vi "SysDef.SimpleSave.vi"(8 "error in (no error)":errorcluster, 11 "ID":u64) -> (0 "error out":errorcluster, 3 "ID out":u64)   [LabVIEW 2015, in "System Definition Utilities.lvlib"]
uses:
  System Definition Utilities.lvlib
  _Types/File.DataType.ctl
  _SubVIs/SysDef.Globals.vi
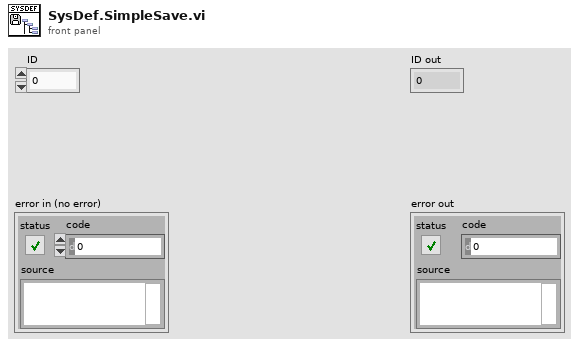
[diagram p1: front panel]
types:
  T1 = typedef "System Definition Utilities.lvlib/SysDef.Export.ctl" = cluster{"Version":string, "Tree":T2[]}
  T2 = typedef "System Definition Utilities.lvlib/TreeItem.ctl" = cluster{"Item Info":T3, "Parent Path":string[], "Properties":T8[]}
  T3 = typedef "System Definition Utilities.lvlib/TreeItem.Info.ctl" = cluster{"Name":string, "Description":string, "GUID":string, "Is Channel":bool, "Channel":T4, "Is Waveform":bool, "Waveform":T6}
  T4 = typedef "Custom Device API.lvlib/Custom Device Channel.ctl" = cluster{"Type":T5, "Units":string, "Default Value":dbl, "Faultable":bool, "Scalable":bool}
  T5 = typedef "Custom Device API.lvlib/Custom Device Channel Type.ctl" = enum16{"Input", "Output"}
  T6 = typedef "Custom Device API.lvlib/Custom Device Waveform.ctl" = cluster{"Data Type":T7, "Units":string}
  T7 = typedef "Custom Device API.lvlib/Custom Device Waveform DataType.ctl" = enum16{"Double", "Complex Double"}
  T8 = typedef "System Definition Utilities.lvlib/TreeItem.Property.ctl" = cluster{"Name":string, "Type":i32, "Value":variant}
  T9 = enum16{"open", "replace", "create", "open or create", "replace or create", "replace or create with confirmation"}
  T10 = typedef "System Definition Utilities.lvlib/File.DataType.ctl" = cluster{"Version":string, "Data":variant}
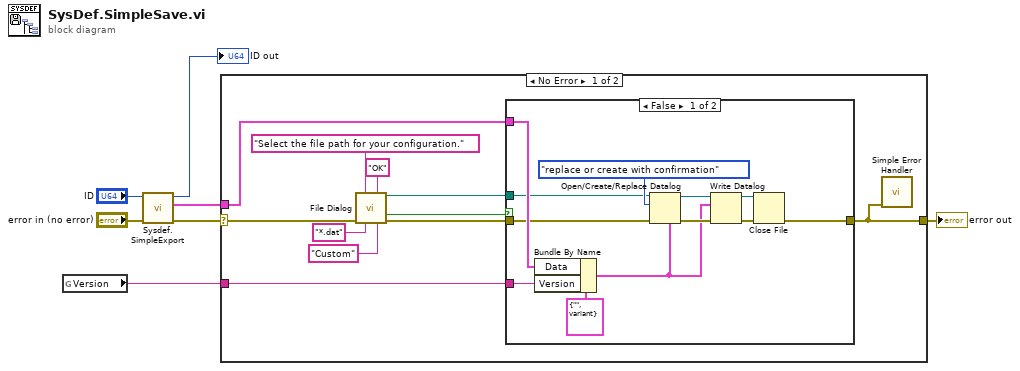
[diagram p0: block diagram]
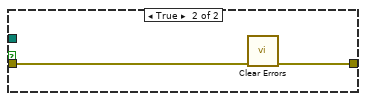
[diagram p2: hidden frame]
diagram:
  n1 = global read "SysDef.Globals.vi" "Version"() -> (w1:string)
  n2 = call "Sysdef.SimpleExport.vi"("error in (no error)"="error in (no error)", "ID"="ID") -> ("error out"=w7:errorcluster, "Export"=w6:T1, "ID out"=→"ID out":u64)  [unwired: 7 in]
  n3 = case shown="No Error" w7 {
    selector: w7 -> [w14 w33]
    tunnel: [w8 w33] -> w2
    tunnel: w6 -> [w10 _]
    tunnel: w1 -> [w9 _]
    frame No Error {
      n4 = call "File Dialog"("prompt"="Select the file path for your configuration.", "button label"="OK", "error in"=w14, "pattern (all files)"="*.dat", "pattern label"="Custom") -> ("selected path"=w11:path, "cancelled"=w13:bool, "error out"=w12:errorcluster)  [unwired: 7 in, 1 out]
      n5 = case shown="False" w13 {
        tunnel: [w19 w31] -> w8
        tunnel: w12 -> [w26 w32]
        tunnel: w11 -> [w25 _]
        tunnel: w10 -> [w28 _]
        tunnel: w9 -> [w30 _]
        frame False {
          n6 = Bundle By Name(cluster=T10 {"Version"="", "Data"=variant}, "Data"=w28, "Version"=w30) -> (w22:T10)
          n7 = Open/Create/Replace Datalog(5:w22, 8:w26, 10:T9."replace or create with confirmation" ("operation (0:open)"), 11:w25) -> (0:w24:errorcluster, 3:w23:refnum<k1>)  [unwired: 2 in, 1 out]
          n8 = Write Datalog(4:w24, 6:w22, 7:w23) -> (0:w21:errorcluster, 3:w20:refnum<k1>)
          n9 = Close File(refnum=w20, error in=w21) -> (error out=w19:errorcluster)  [unwired: 1 out]
        }
        frame True {
          n10 = call <vilib>:"Clear Errors.vi"("error in (no error)"=w32) -> ("error out"=w31:errorcluster)  [unwired: 5 in, 1 out]
        }
      }
      n11 = call <vilib>:"Simple Error Handler.vi"("error in (no error)"=w8) -> ()  [unwired: 4 in, 5 out]
    }
    frame Error {
    }
  }
  "error out" <- w2
